vi "SigSyn (G3)-Get Valid Sequence Variables (1D).vi"(9 "Endpoint Config":T1[](array[typedef]), 11 "StimChans":T4[](array[typedef]) {"Filter"."Stages"."IIR Filter"."Forward Coefficients" format="%.4f"; "Filter"."Stages"."IIR Filter"."Reverse Coefficients" format="%.4f"}) -> (3 "Valid Params":string[](array[string]))   [LabVIEW 2020]
uses:
  XControls/Stimulus Channel (G3)/Full Stimulus Channel Data.ctl
  XControls/Waveform XControls/Waveform (G3)/Waveform Data.ctl
  Waveform VIs/Waveform Enum (V3).ctl
  XControls/Waveform XControls/Tone (G3)/Tone.Properties.ctl
  Waveform VIs/Pulse Train VIs/Pulse Train Params.ctl
  Waveform VIs/Pulse Train VIs/Pulse Polarity.ctl
  Waveform VIs/Pulse Train VIs/PT-Continuous State.ctl
  Waveform VIs/Noise VIs/Noise (G3).ctl
  Waveform VIs/Noise VIs/Noise (G3).Properties.ctl
  Waveform VIs/Noise VIs/Noise (G3).Data.ctl
  Waveform VIs/File VIs/StimFile-Params.ctl
  Waveform VIs/FM Sweep VIs/FM Sweep Params.ctl
  Waveform VIs/Chirp Train VIs/Chirp Train.ctl
  Waveform VIs/Chirp Train VIs/Chirp Train Params.ctl
  Waveform VIs/Complex Tone VIs/CT-Params.ctl
  Waveform VIs/Complex Tone VIs/CT-Phase Enum.ctl
  Waveform VIs/Complex Tone VIs/CT-Runtime Data.ctl
  XControls/Waveform XControls/FM Tone/Data.ctl
  XControls/Waveform XControls/Vowel/Vowel.Properties.ctl
  Waveform VIs/Ramp VIs/Ramp.Properties.ctl
  XControls/Filter (G3)/Filter Data.ctl
  XControls/Filter (G3)/Filter Type.ctl
  Filter VIs/Filter-Bandwidth Units.ctl
  Controls/Burst XCtl/Burst Data.ctl
  XControls/Level (G3)/Level Data.ctl
  XControls/Level (G3)/Level Units (G3).ctl
  XControls/Advanced Options (G3)/Advanced Options (G3).ctl
  Modulation VIs/SAM VIs/SAM Params.ctl
  Typedefs/Destination.ctl
  Calibration VIs/Endpoint VIs/LV Source/Endpoint-Spec.ctl
  Calibration VIs/Endpoint VIs/LV Source/Endpoint-Modality.ctl
  Calibration VIs/Endpoint VIs/LV Source/Endpoint-Laterality.ctl
  Controls/Waveform XCtl/Waveform Enum.ctl
  XControls/Filter (G3)/Filter (G3).xctl
  XControls/Level (G3)/Level (G3).xctl
  Controls/Burst XCtl/Burst Control.xctl
  XControls/Waveform XControls/Waveform (G3)/Waveform (G3).xctl
  XControls/Advanced Options (G3)/Advanced Options (G3).xctl
  XControls/Stimulus Channel (G3)/Stimulus Channel (G3).xctl
  XControls/Waveform XControls/Tone (G3)/Tone (G3).xctl
  XControls/Waveform XControls/FM Tone/FM Tone.xctl
  XControls/Waveform XControls/Vowel/Vowel.xctl
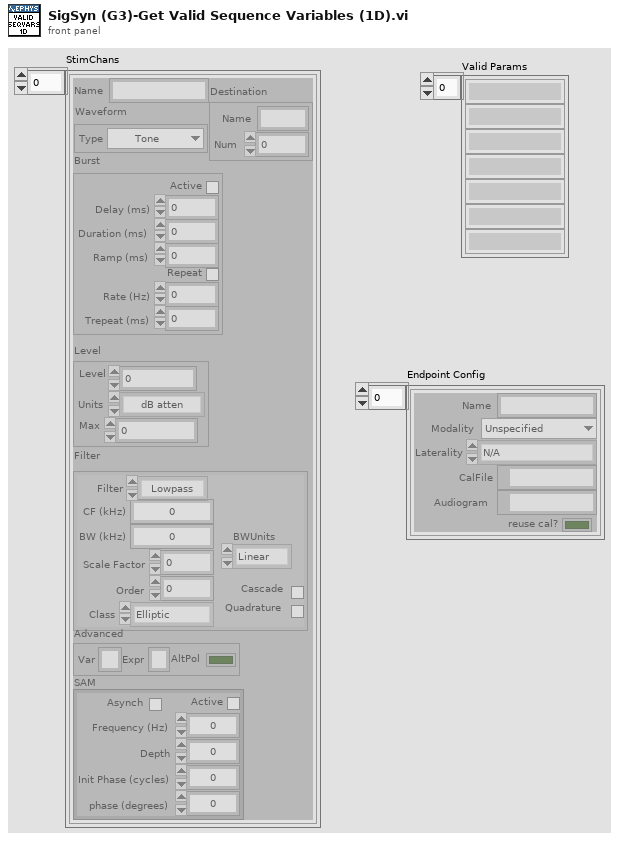
[diagram p1: front panel]
types:
  T1 = typedef "Endpoint-Spec.ctl" = cluster{"Name":string, "Modality":T2, "Laterality":T3, "CalFile":path, "Audiogram":path, "reuse cal?":bool}
  T2 = typedef "Endpoint-Modality.ctl" = enum16{"Unspecified", "Acoustic", "Electric", "Optical"}
  T3 = typedef "Endpoint-Laterality.ctl" = enum16{"N/A", "Right", "Left"}
  T4 = typedef "Stimulus Channel (G3).xctl/Full Stimulus Channel Data.ctl" = cluster{"Waveform":T5, "Filter":T24, "Burst":T27, "Level":T28, "Name":string, "Advanced":T30, "SAM":T31, "Destination":T32}
  T5 = typedef "Waveform (G3).xctl/Waveform Data.ctl" = cluster{"Type":T6, "Tone":T7, "Pulse Train":T8, "Noise":T11, "File":T14, "FMSweep":T15, "Chirp Train":T16, "Complex Tone":cluster{"Params":T18, "Data":T20}, "FM":T21, "Vowel":T22, "Ramp":T23}
  T6 = typedef "Waveform Enum (V3).ctl" = enum16{"OFF", "Tone", "Noise", "Pulse Train", "File", "FM Sweep", "Chirp Train", "Complex Tone", "FM Tone", "Vowel", "Ramp"}
  T7 = typedef "Tone (G3).xctl/Tone.Properties.ctl" = cluster{"Frequency (kHz)":dbl, "Phase (cycles)":dbl, "Random phase":bool}
  T8 = typedef "Pulse Train Params.ctl" = cluster{"Pulse width (us)":dbl, "Pulse rate (Hz)":dbl, "Gap (ms)":dbl, "Polarity":T9, "PT State":T10, "Asynch":bool}
  T9 = typedef "Pulse Polarity.ctl" = enum16{"POS", "NEG", "POS-NEG", "NEG-POS"}
  T10 = typedef "PT-Continuous State.ctl" = cluster{"Template":dbl[], "Nperiod":i32, "Index":i32, "Pulse Rate (Hz)":dbl, "Phase (cycles)":dbl, "Noff":i32}
  T11 = typedef "Noise (G3).ctl" = cluster{"Properties":T12, "Data":T13}
  T12 = typedef "Noise (G3).Properties.ctl" = cluster{"InvFilt":bool, "Aweight":bool, "Seed":i32, "Tokens":i32, "Brickwall":bool}
  T13 = typedef "Noise (G3).Data.ctl" = cluster{"TokenNum":i32}
  T14 = typedef "StimFile-Params.ctl" = cluster{"Filename":path, "Signal":dbl[], "Channel":i32, "stream":bool, "offset":i32, "nreps":i32, "loops":i32, "Randomize":bool, "order":i32[], "Seed":i32, "Tokens":i32}
  T15 = typedef "FM Sweep Params.ctl" = cluster{"Rate (oct/s)":dbl, "Fmin (Hz)":dbl, "Fmax (Hz)":dbl, "Ramp (ms)":dbl, "Linear":bool}
  T16 = typedef "Chirp Train.ctl" = cluster{"Params":T17, "Data":cluster{"WF":dbl[]}}
  T17 = typedef "Chirp Train Params.ctl" = cluster{"Fmin (kHz)":dbl, "Fmax (kHz)":dbl, "Compensate":bool, "Duration (ms)":dbl}
  T18 = typedef "CT-Params.ctl" = cluster{"F0 (Hz)":dbl, "Band":cluster{"Flow (Hz)":dbl, "Fhigh (Hz)":dbl}, "Phase":T19, "Min F0 (Hz)":dbl, "Max F0 (Hz)":dbl, "ContinRandPhase":bool, "Max peak factor":dbl, "Max mod depth":dbl, "MinHarmNum":i32, "MaxHarmNum":i32, "Level Mode":enum16{"per component", "overall rms"}, "% jitter":dbl}
  T19 = typedef "CT-Phase Enum.ctl" = enum16{"Cosine", "Random", "Alternating"}
  T20 = typedef "CT-Runtime Data.ctl" = cluster{"Ncomp":i32, "MinHarm":i32, "Phase":dbl[], "Amplitude":dbl[], "Npts/frame":i32, "Last F0":dbl, "Fmin":dbl, "Fmax":dbl, "Lslope":dbl, "randphase":bool, "overall rms":bool, "fmult":dbl[], "jittered":bool}
  T21 = typedef "FM Tone.xctl/Data.ctl" = cluster{"Carrier (kHz)":dbl, "ModRate (Hz)":dbl, "Depth (Hz)":dbl, "Phase (cycles)":dbl}
  T22 = typedef "Vowel.xctl/Vowel.Properties.ctl" = cluster{"Freqs":string, "Set level":enum16{"Total", "Per component"}, "Freq":dbl[], "weights":dbl[]}
  T23 = typedef "Ramp.Properties.ctl" = cluster{"Duration (ms)":dbl}
  T24 = typedef "Filter (G3).xctl/Filter Data.ctl" = cluster{"Type":T25, "CF (kHz)":dbl, "BW (kHz)":dbl, "Cascade":bool, "Quadrature":bool, "Scale Factor":dbl, "Stages":cluster{"IIR Filter":cluster{"filter structure":enum32{"IIR 2nd Order", "IIR 4th Order"}, "Reverse Coefficients":dbl[], "Forward Coefficients":dbl[]}, "State":dbl[]}[], "Class":enum16{"Elliptic", "Butterworth"}, "Order":i32, "BWUnits":T26}
  T25 = typedef "Filter (G3).xctl/Filter Type.ctl" = enum16{"OFF", "Lowpass", "Highpass", "Bandpass", "Bandstop"}
  T26 = typedef "Filter-Bandwidth Units.ctl" = enum16{"Linear", "Octaves", "Min-Max"}
  T27 = typedef "Burst Control.xctl/Burst Data.ctl" = cluster{"Active":bool, "Delay (ms)":dbl, "Duration (ms)":dbl, "Ramp (ms)":dbl, "Rate (Hz)":dbl, "Trepeat (ms)":dbl, "Repeat":bool}
  T28 = typedef "Level (G3).xctl/Level Data.ctl" = cluster{"Level":dbl, "Units":T29, "Max":dbl, "Data":cluster{"Multiplier":dbl, "Cal File":path, "Cal":cluster{"Freq (Hz)":dbl[], "Mag (dB SPL)":dbl[], "Phase (deg)":dbl[]}, "audiogram":path}}
  T29 = typedef "Level (G3).xctl/Level Units (G3).ctl" = enum16{"dB atten", "dB SPL", "dB re 1 Vrms", "dB V/Hz½", "mW", "dB HL", "Volts", "dB mW"}
  T30 = typedef "Advanced Options (G3).xctl/Advanced Options (G3).ctl" = cluster{"AltPol":bool, "Var":string, "Expr":string}
  T31 = typedef "SAM Params.ctl" = cluster{"Active":bool, "Frequency (Hz)":dbl, "Depth":dbl, "Init Phase (cycles)":dbl, "phase (degrees)":dbl, "Asynch":bool}
  T32 = typedef "Destination.ctl" = cluster{"Name":string, "Num":i32}
  T33 = typedef "Waveform Enum.ctl" = enum16{"OFF", "Tone", "Noise", "Pulse Train", "File", "FM Sweep", "Chirp Train", "Complex Tone", "FM Tone", "Moving Ripple"}
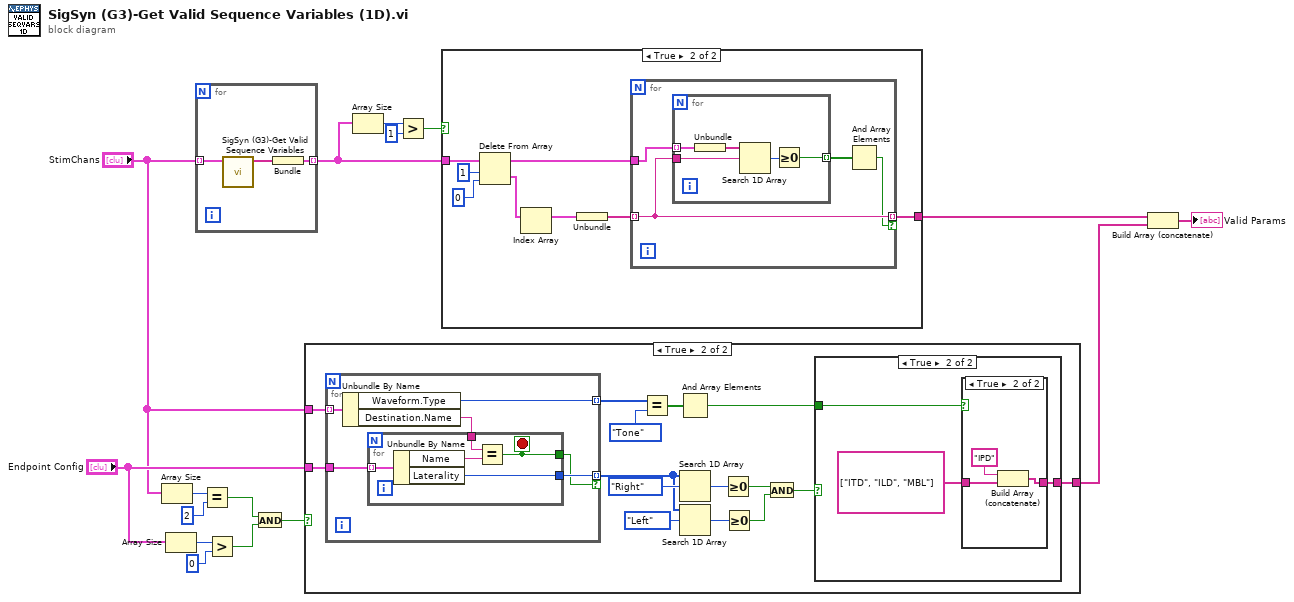
[diagram p0: block diagram]
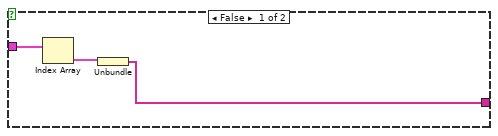
[diagram p5: hidden frame]
diagram:
  n1 = Array Size(array="StimChans") -> (size(s)=w11:i32)
  n2 = Array Size(array="Endpoint Config") -> (size(s)=w9:i32)
  n3 = for {
    tunnel: "StimChans" -> [w19] mode=indexing
    tunnel: [w17] -> w16 mode=indexing
    n4 = call "SigSyn (G3)-Get Valid Sequence Variables.vi"("Stimulus"=w19) -> ("Valid Params"=w18:string[])  [unwired: 10 in]
    n5 = Bundle("Valid Params"=w18) -> (w17:cluster{"Valid Params":string[]})  [unwired: 1 in]
  }
  n6 = Equal?(x=w11, y=2) -> (x = y?=w7:bool)
  n7 = Greater?(x=w9, y=0) -> (0:w6:bool)
  n8 = And(x=w7, y=w6) -> (x .and. y?=w5:bool)
  n9 = case shown="True" w5 {
    tunnel: "Endpoint Config" -> [_ w34]
    tunnel: "StimChans" -> [_ w33]
    tunnel: [_ w20] -> w1
    frame False {
    }
    frame True {
      n10 = for {
        tunnel: w34 -> [w46]
        tunnel: w33 -> [w47] mode=indexing
        tunnel: [w44] -> w31 mode=indexing if=w43
        tunnel: [w42] -> w24 mode=indexing
        n11 = Unbundle By Name(w47) -> ("Waveform.Type"=w42:T6, "Destination.Name"=w45:string)
        n12 = for {
          tunnel: w46 -> [w52] mode=indexing
          tunnel: w45 -> [w50]
          tunnel: [w49] -> w44
          tunnel: [w48] -> w43
          stop <- w48 stop-if-true
          n13 = Unbundle By Name(w52) -> ("Name"=w51:string, "Laterality"=w49:T3)
          n14 = Equal?(x=w50, y=w51) -> (x = y?=w48:bool)
        }
      }
      n15 = Equal?(x=w24, y=Waveform_Enum."Tone" ("Waveform.Type")) -> (x = y?=w22:bool[])
      n16 = And Array Elements(Boolean array=w22) -> (logical AND=w21:bool)
      n17 = Search 1D Array(1D array=w31, element=Endpoint-Laterality."Right") -> (index of element=w29:i32)  [unwired: 1 in]
      n18 = Search 1D Array(1D array=w31, element=Endpoint-Laterality."Left") -> (index of element=w28:i32)  [unwired: 1 in]
      n19 = Greater Or Equal To 0?(x=w29) -> (x >= 0?=w27:bool)
      n20 = Greater Or Equal To 0?(x=w28) -> (x >= 0?=w26:bool)
      n21 = And(x=w27, y=w26) -> (x .and. y?=w25:bool)
      n22 = case shown="True" w25 {
        tunnel: w21 -> [_ w37]
        tunnel: [_ w35] -> w20
        frame False {
        }
        frame True {
          n23 = case shown="True" w37 {
            tunnel: string[] ["ITD", "ILD", "MBL"] -> [w38 w41]
            tunnel: [w38 w40] -> w35
            frame False {
            }
            frame True {
              n24 = Build Array (concatenate)("IPD", w41) -> (w40:string[])
            }
          }
        }
      }
    }
  }
  n25 = Array Size(array=w16) -> (size(s)=w15:i32)
  n26 = Greater?(x=w15, y=1) -> (0:w13:bool)
  n27 = case shown="True" w13 {
    tunnel: w16 -> [w54 w57]
    tunnel: [w53 w56] -> w12
    frame False {
      n28 = Index Array(array=w54) -> (element=w55:cluster{"Valid Params":string[]})  [unwired: 1 in]
      n29 = Unbundle(w55) -> ("Valid Params"=w53:string[])
    }
    frame True {
      n30 = Delete From Array(array=w57, length=1, index=0) -> (deleted portion=w62:cluster{"Valid Params":string[]}[], array with subset deleted=w61:cluster{"Valid Params":string[]}[])
      n31 = Index Array(array=w62) -> (element=w60:cluster{"Valid Params":string[]})  [unwired: 1 in]
      n32 = Unbundle(w60) -> ("Valid Params"=w58:string[])
      n33 = for {
        tunnel: w58 -> [w66] mode=indexing
        tunnel: w61 -> [w67]
        tunnel: [w66] -> w56 mode=indexing if=w64
        n34 = for {
          tunnel: w67 -> [w72] mode=indexing
          tunnel: w66 -> [w70]
          tunnel: [w68] -> w65 mode=indexing
          n35 = Unbundle(w72) -> ("Valid Params"=w71:string[])
          n36 = Search 1D Array(1D array=w71, element=w70) -> (index of element=w69:i32)  [unwired: 1 in]
          n37 = Greater Or Equal To 0?(x=w69) -> (x >= 0?=w68:bool)
        }
        n38 = And Array Elements(Boolean array=w65) -> (logical AND=w64:bool)
      }
    }
  }
  n39 = Build Array (concatenate)(w12, w1) -> (→"Valid Params":string[])
